vi "sedSpectrometer_getEvent_summaryState.vi"(8 "error in (no error)":errorcluster, 11 "logevent_summaryState_Ctl":T1) -> (0 "error out":errorcluster, 2 "function return":i32, 3 "logevent_summaryState_Ctl out":T1)   [LabVIEW 2016, in "SALLV_sedSpectrometer.lvlib"]
doc: "int sedSpectrometer_shm_getEvent_summaryStateLV(sedSpectrometer_logevent_summaryStateLV *logevent_summaryState_Ctl );"
uses:
  SALLV_sedSpectrometer.lvlib
  DataTypes/logevent_summaryState.ctl
  SALLV_sedSpectrometer.so
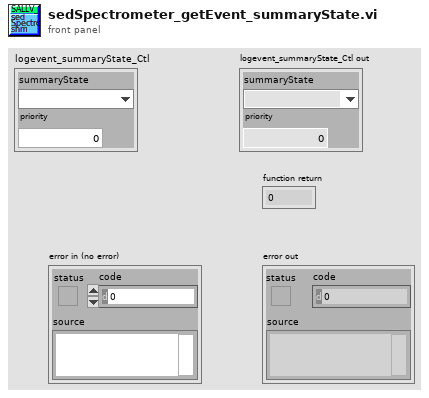
[diagram p1: front panel]
types:
  T1 = typedef "SALLV_sedSpectrometer.lvlib/logevent_summaryState.ctl" = cluster{"summaryState":enum32{"", "DisabledState", "EnabledState", "FaultState", "OfflineState", "StandbyState"}, "priority":i32}
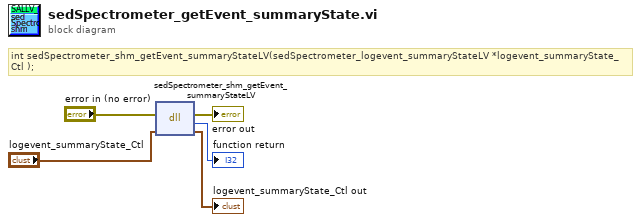
[diagram p0: block diagram]
diagram:
  # "int sedSpectrometer_shm_getEvent_summaryStateLV(sedSpectrometer_logevent_summaryStateLV *logevent_summaryState_Ctl );"
  n1 = dll-call lib="home/harini/tcs/ts_sedspectrometer/ts_sallv_sedspectrometer/SALLV_sedSpectrometer.*" fn="sedSpectrometer_shm_getEvent_summaryStateLV"(error in="error in (no error)", "logevent_summaryState_Ctl"="logevent_summaryState_Ctl") -> (error out=→"error out":errorcluster, →"function return":i32, "logevent_summaryState_Ctl"=→"logevent_summaryState_Ctl out":T1)  [unwired: 2 in, 1 out]
